vi "verify websocket conditions.vi"(10 "HTTP protocol version":T1, 11 "HTTP method":T2) -> (0 "error out":errorcluster)   [LabVIEW 2019, in "WebSocket Server Toolkit.lvlib"]
uses:
  WebSocket Server Toolkit.lvlib
  types/HTTP Request Method.ctl
  types/HTTP Protocol Version.ctl
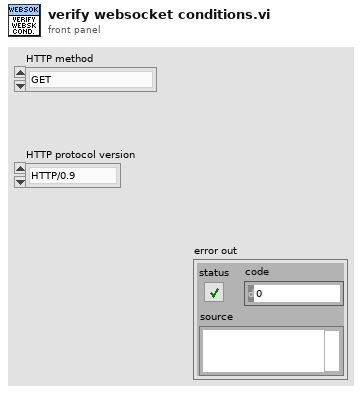
[diagram p1: front panel]
types:
  T1 = typedef "WebSocket Server Toolkit.lvlib/HTTP Protocol Version.ctl" = enum16{"HTTP/0.9", "HTTP/1.0", "HTTP/1.1", "HTTP/2.0", "HTTP/3.0"}
  T2 = typedef "WebSocket Server Toolkit.lvlib/HTTP Request Method.ctl" = enum16{"GET", "HEAD", "POST", "PUT", "DELETE", "CONNECT", "OPTIONS", "TRACE", "PATCH"}
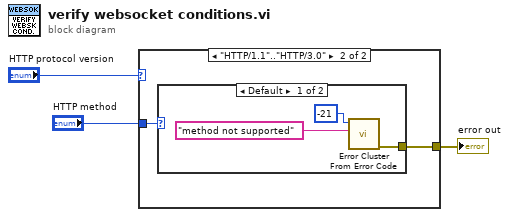
[diagram p0: block diagram]
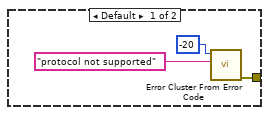
[diagram p2: hidden frame]
diagram:
  n1 = case shown="\"HTTP/1.1\"..\"HTTP/3.0\"" "HTTP protocol version" {
    tunnel: [w4 w7] -> w2
    tunnel: "HTTP method" -> [_ w8]
    frame Default {
      n2 = call <vilib>:"Error Cluster From Error Code.vi"("error message (\"\")"="protocol not supported" ("error message (\"\")"), "error code (0)"=-20) -> ("error out"=w4:errorcluster)  [unwired: 7 in]
    }
    frame "HTTP/1.1".."HTTP/3.0" {
      n3 = case shown="Default" w8 {
        tunnel: [w9 _] -> w7
        frame Default {
          n4 = call <vilib>:"Error Cluster From Error Code.vi"("error message (\"\")"="method not supported" ("error message (\"\")"), "error code (0)"=-21) -> ("error out"=w9:errorcluster)  [unwired: 7 in]
        }
        frame "GET" {
        }
      }
    }
  }
  "error out" <- w2
